vi "ReadWrite.ProcessData.Write.vi"(8 "error in":errorcluster, 9 "Offset":i32, 10 "Values":dbl[](array[numeric]), 11 "ReadWrite in":refnum<class "ReadWrite.lvclass">) -> (0 "error out":errorcluster, 3 "ReadWrite out":refnum<class "ReadWrite.lvclass">)   [LabVIEW 2024, in "VS Plugin Inline Async API.lvlib" / "ReadWrite.lvclass"]
uses:
  ReadWrite.lvclass
  ReadWrite.lvclass/ReadWrite.ctl
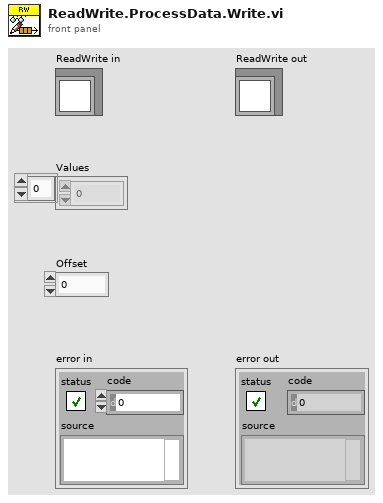
[diagram p1: front panel]
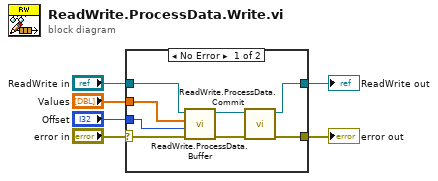
[diagram p0: block diagram]
diagram:
  n1 = case shown="No Error" "error in" {
    selector: "error in" -> [w14 w16]
    tunnel: [w12 w16] -> w5
    tunnel: [w7 w15] -> w1
    tunnel: "ReadWrite in" -> [w9 w15]
    tunnel: "Values" -> [w10 _]
    tunnel: "Offset" -> [w11 _]
    frame No Error {
      n2 = call "ReadWrite.ProcessData.Buffer.vi"("error in"=w14, "Offset"=w11, "Values"=w10, "ReadWrite in"=w9) -> ("error out"=w13:errorcluster, "ReadWrite out"=w8:refnum<class "ReadWrite.lvclass">)  [unwired: 6 in]
      n3 = call "ReadWrite.ProcessData.Commit.vi"("error in"=w13, "ReadWrite in"=w8) -> ("error out"=w12:errorcluster, "ReadWrite out"=w7:refnum<class "ReadWrite.lvclass">)  [unwired: 8 in]
    }
    frame Error {
    }
  }
  "error out" <- w5
  "ReadWrite out" <- w1
